vi "Round with options.vi"(1 "Round mode selection":u16(ring) items=["Round to nearest", "Round to -inf", "Round to +inf"], 2 "Numeric in":dbl format="%.6f", 3 "Num array in":dbl[](array[numeric]) format="%.6f", 4 "No.of digits\nto round to":i16=2) -> (14 "Numeric out":dbl format="%.6f", 15 "Num array out":dbl[](array[numeric]) format="%.6f")   [LabVIEW 2020]
doc: "Rounds Numeric in and Num array according to No. of digits to round to and Round mode selection."
panel:
  # "Rounds \"Numeric in\" and \"Num array\" according to \"No. of digits \nto round to\" and \"Round mode selection\"."
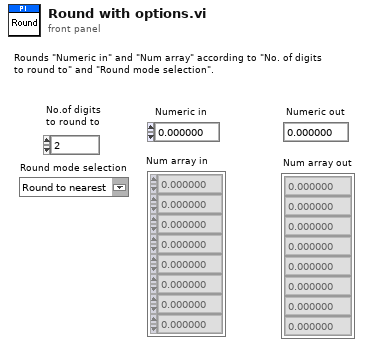
[diagram p1: front panel]
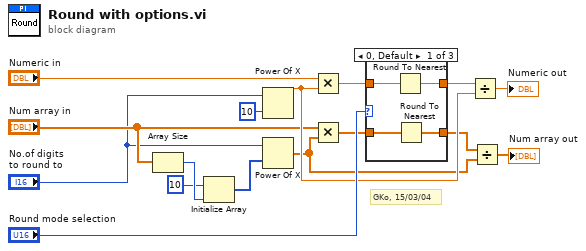
[diagram p0: block diagram]
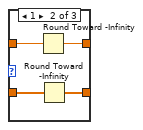
[diagram p2: hidden frame]
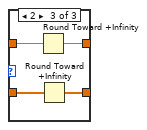
[diagram p3: hidden frame]
diagram:
  # "GKo, 15/03/04"
  n1 = Array Size(array="Num array in") -> (size(s)=w6:i32)
  n2 = Initialize Array(i16 10 ("x"), w6) -> (w3:i16[])
  n3 = Power Of X(1:i16 10 ("x"), 2:"No.of digits\nto round to") -> (0:w10:dbl)
  n4 = Power Of X(1:w3, 2:"No.of digits\nto round to") -> (0:w1:dbl[])
  n5 = Multiply(x="Numeric in", y=w10) -> (x*y=w14:dbl)
  n6 = Multiply(x="Num array in", y=w1) -> (x*y=w2:dbl[])
  n7 = case shown="0, Default" "Round mode selection" {
    tunnel: w14 -> [w20 w24 w28]
    tunnel: w2 -> [w19 w23 w27]
    tunnel: [w18 w22 w26] -> w13
    tunnel: [w17 w21 w25] -> w8
    frame 0, Default {
      n8 = Round To Nearest(number=w20) -> (nearest integer value=w18:dbl)
      n9 = Round To Nearest(number=w19) -> (nearest integer value=w17:dbl[])
    }
    frame 1 {
      n10 = Round Toward -Infinity(1:w24) -> (0:w22:dbl)
      n11 = Round Toward -Infinity(1:w23) -> (0:w21:dbl[])
    }
    frame 2 {
      n12 = Round Toward +Infinity(x=w28) -> (ceil(x): smallest int >= x=w26:dbl)
      n13 = Round Toward +Infinity(x=w27) -> (ceil(x): smallest int >= x=w25:dbl[])
    }
  }
  n14 = Divide(x=w13, y=w10) -> (x/y=→"Numeric out":dbl)
  n15 = Divide(x=w8, y=w1) -> (x/y=→"Num array out":dbl[])
